vi "ATF-PPSU Device list.vi"(7 "Enum":enum16{"Read", "Write"}(ring), 8 "error in":errorcluster, 11 "Device information array":string[](array[string])) -> (0 "error out":errorcluster, 3 "Device information arrayR":string[](array[string]))   [LabVIEW 2022 SP3]
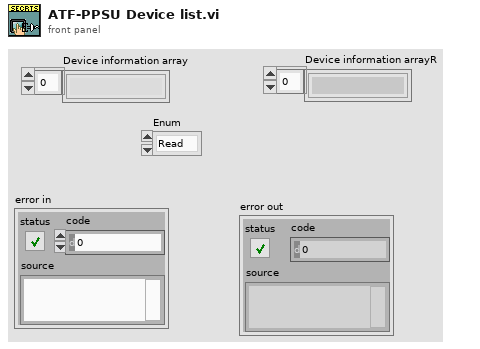
[diagram p1: front panel]
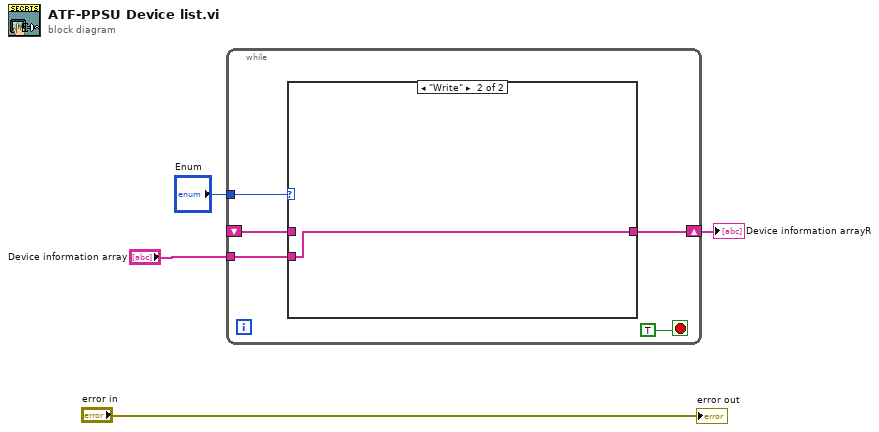
[diagram p0: block diagram]
diagram:
  n1 = while {
    tunnel: "Enum" -> [w9]
    tunnel: "Device information array" -> [w7]
    shift-right: [w6] -> w1
    shift-left: _ -> [w5]
    stop <- TRUE stop-if-true
    n2 = case shown="\"Write\"" w9 {
      tunnel: w7 -> [_ w11]
      tunnel: [w10 w11] -> w6
      tunnel: w5 -> [w10 _]
      frame "Read", Default {
      }
      frame "Write" {
      }
    }
  }
  "Device information arrayR" <- w1
  "error out" <- "error in"
